vi "Translation2d_Create.vi"(10 "Y":dbl, 11 "X":dbl) -> (3 "TRANSLATION":T1 {"Y" format="%14.3f"; "X" format="%14.3f"})   [LabVIEW 2019, in "Trajectory_Library.lvlib"]
doc: "Constructs a Translation2d with the X and Y components equal to the provided values.\n\nRepresents a translation in 2d space. This object can be used to represent a point or a vector.\n\nThis assumes that you are using conventional mathematical axes. When the robot is placed on the origin, facing toward the X direction, moving forward increases the X, whereas moving to the left increases the Y.\n\nParameters:\n - X - The x component of the translation.\n - Y - The y component of the translation.\n\nReturns\n - TRANSLATION - The TRANSLATION data structure"
uses:
  Trajectory_Library.lvlib
  TRANSLATION2D.ctl
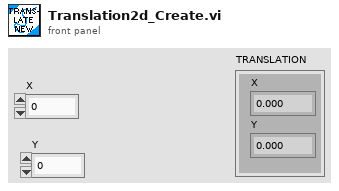
[diagram p1: front panel]
types:
  T1 = typedef "Trajectory_Library.lvlib/TRANSLATION2D.ctl" = cluster{"X":dbl, "Y":dbl}
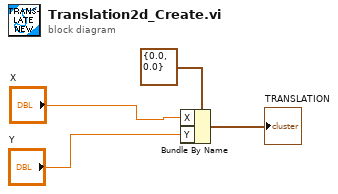
[diagram p0: block diagram]
diagram:
  n1 = Bundle By Name(cluster=T1 {"X"=0.0, "Y"=0.0} ("TRANSLATION"), "X"="X", "Y"="Y") -> (→"TRANSLATION":T1)
